vi "Proxy template.vi"(8 "Globals":refnum<data-value>, 9 "E-Stop":refnum<user-event>, 10 "Response":refnum<user-event>, 11 "RequestMQ":refnum<queue>) -> ()   [LabVIEW 2020, in "Module.lvlib" / "Module.lvclass"]
uses:
  Module.lvclass
  RPC/TypeDefs/Request.ctl
  RPC/TypeDefs/Response.ctl
  Module.lvclass/Module.ctl
  RPC.lvlib
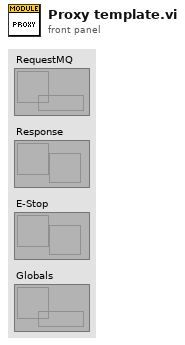
[diagram p1: front panel]
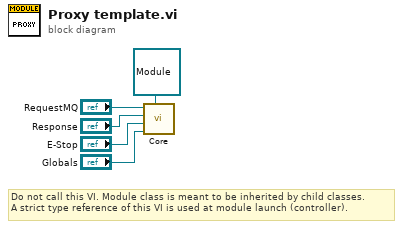
[diagram p0: block diagram]
diagram:
  # "Do not call this VI. Module class is meant to be inherited by child classes.\nA strict type reference of this VI is used at module launch (controller)."
  n1 = call-dynamic "Core.vi"("ObjRef"=refnum<class "Module.lvclass"> refnum ("Module.lvlib:Module.lvclass"), "Globals"="Globals", "E-Stop"="E-Stop", "Response"="Response", "RequestMQ"="RequestMQ") -> ()  [unwired: 7 in]
